vi "FTW-Test-Regex-BasicUsage.vi"() -> (0 "Test Result":errorcluster)   [LabVIEW 2014]
uses:
  src/core/error/FTW-ERR-Assert-DeveloperError.vi
  src/core/error/FTW-ERR-ThrowError.vi
  src/core/error/FTW-ERR-CallChain.vi
  src/core/string/FTW-STR-ReplaceWhitespace.vi
  src/core/regex/FTW-Regex.lvclass
panel:
  out "Callouts":T1(array[cluster])
  out "Array 2":string[](array[string])
  out "Numeric":i32
  out "Submatches":i32[](array[numeric])
  out "Array":i32[](array[numeric])
  out "Capture Groups":string[](array[string])
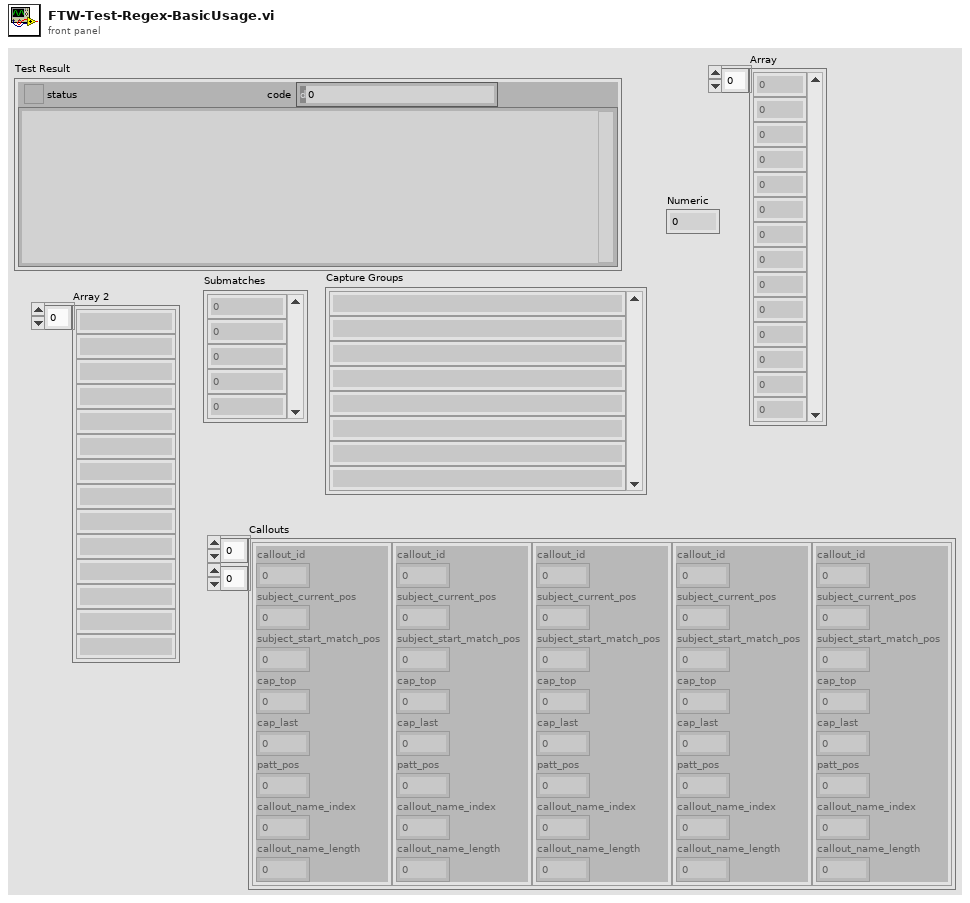
[diagram p1: front panel]
types:
  T1 = cluster{"callout_id":i32, "subject_current_pos":i32, "subject_start_match_pos":i32, "cap_top":i32, "cap_last":i32, "patt_pos":i32, "callout_name_index":i32, "callout_name_length":i32}[][]
  T2 = cluster{"callout_id":i32, "subject_current_pos":i32, "subject_start_match_pos":i32, "cap_top":i32, "cap_last":i32, "patt_pos":i32, "callout_name_index":i32, "callout_name_length":i32}[]
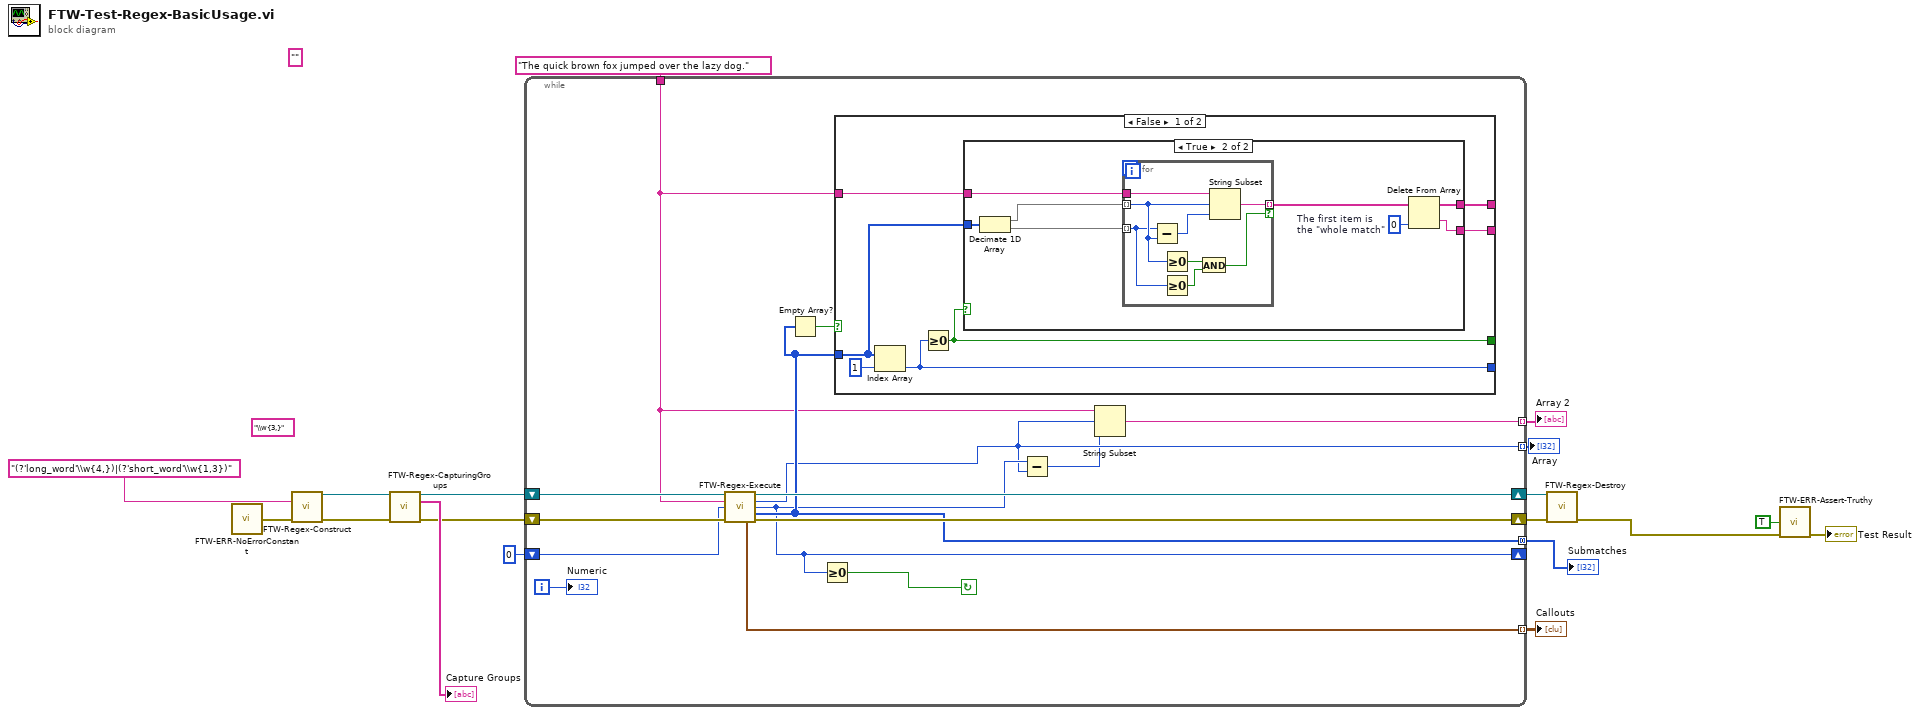
[diagram p0: block diagram]
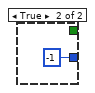
[diagram p3: hidden frame]
diagram:
  (unwired) "" ("Regular Expression")
  (unwired) "\\w{3,}" ("Regular Expression")
  n1 = call "FTW-ERR-NoErrorConstant.vi"() -> ("no error"=w14:errorcluster)
  n2 = call "FTW-Regex-Construct.vi"("Regular Expression"="(?'long_word'\\w{4,})|(?'short_word'\\w{1,3})", "error in"=w14) -> ("Regex"=w17:refnum<class "FTW-Regex.lvclass">, "error out"=w15:errorcluster)  [unwired: 12 in]
  n3 = call "FTW-Regex-CapturingGroups.vi"("Regex"=w17, "error in"=w15) -> ("Regex out"=w13:refnum<class "FTW-Regex.lvclass">, "Capture Groups"=→"Capture Groups":string[], "error out"=w11:errorcluster)  [unwired: 11 in]
  n4 = while {
    shift-right: [w32] -> w12
    shift-left: w13 -> [w33]
    shift-right: [w30] -> w10
    shift-left: w11 -> [w31]
    tunnel: [w22] -> w8 mode=indexing
    tunnel: "The quick brown fox jumped over the lazy dog." ("Subject String") -> [w24]
    shift-right: [w23] -> _
    shift-left: 0 ("Offset after Match") -> [w29]
    tunnel: [w25] -> w4 mode=concatenating
    tunnel: [w20] -> w2 mode=indexing
    tunnel: [w19] -> w1 mode=indexing
    i -> [w27]
    stop <- w28 continue-if-true
    n5 = call "FTW-Regex-Execute.vi"("Regex"=w33, "Subject String"=w24, "Starting Offset"=w29, "error in"=w31) -> ("Regex out"=w32:refnum<class "FTW-Regex.lvclass">, "Whole Match Begin"=w22:i32, "Offset after Match"=w23:i32, "Submatches"=w25:i32[], "Callouts"=w19:T2, "error out"=w30:errorcluster)  [unwired: 6 in]
    n6 = Empty Array?(array=w25) -> (empty?=w26:bool)
    n7 = Greater Or Equal To 0?(x=w23) -> (x >= 0?=w28:bool)
    n8 = case shown="False" w26 {
      tunnel: [w40 _] -> _
      tunnel: [w39 _] -> _
      tunnel: [w37 -1] -> _
      tunnel: [w36 _] -> _
      tunnel: w24 -> [w35 _]
      tunnel: w25 -> [w34 _]
      frame False {
        n9 = Index Array(array=w34, index=1) -> (element=w37:i32)
        n10 = Greater Or Equal To 0?(x=w37) -> (x >= 0?=w36:bool)
        n11 = case shown="True" w36 {
          tunnel: w35 -> [_ w48]
          tunnel: [_ w44] -> w40
          tunnel: [_ w43] -> w39
          tunnel: w34 -> [_ w41]
          frame False {
          }
          frame True {
            w45 = 0  # The first item is the "whole match"
            n12 = Decimate 1D Array(w41) -> (w47:i32[], w42:i32[])
            n13 = for {
              tunnel: w48 -> [w56]
              tunnel: [w55] -> w46 mode=indexing if=w50
              tunnel: w47 -> [w53] mode=indexing
              tunnel: w42 -> [w49] mode=indexing
              n14 = Subtract(x=w49, y=w53) -> (x-y=w54:i32)
              n15 = Greater Or Equal To 0?(x=w53) -> (x >= 0?=w52:bool)
              n16 = Greater Or Equal To 0?(x=w49) -> (x >= 0?=w51:bool)
              n17 = And(x=w52, y=w51) -> (x .and. y?=w50:bool)
              n18 = String Subset(string=w56, offset (0)=w53, length (rest)=w54) -> (substring=w55:string)
            }
            n19 = Delete From Array(array=w46, index=w45) -> (deleted portion=w44:string, array with subset deleted=w43:string[])  [unwired: 1 in]
          }
        }
      }
      frame True {
      }
    }
    n20 = Subtract(x=w23, y=w22) -> (x-y=w21:i32)
    n21 = String Subset(string=w24, offset (0)=w22, length (rest)=w21) -> (substring=w20:string)
    "Numeric" <- w27
  }
  "Array" <- w8
  "Submatches" <- w4
  "Array 2" <- w2
  "Callouts" <- w1
  n22 = call "FTW-Regex-Destroy.vi"("Regex"=w12, "error in"=w10) -> ("error out"=w9:errorcluster)  [unwired: 13 in]
  n23 = call "FTW-ERR-Assert-Truthy.vi"("Expected Truthy"=TRUE, "error in"=w9) -> ("error out"=→"Test Result":errorcluster)  [unwired: 13 in]
